vi "Process Event Data.vi"(9 "Event Data":u8[](array[numeric]), 10 "Event Type":u32 format="%.0x", 11 "PS4 Controller in":refnum<class "PS4 Controller.lvclass">) -> (3 "PS4 Controller out":refnum<class "PS4 Controller.lvclass">)   [LabVIEW 2019, in "SDL2 Utility.lvlib" / "PS4 Controller.lvclass"]
uses:
  PS4 Controller.lvclass
  PS4 Controller.lvclass/PS4 Controller.ctl
  LibSDL2 Wrapper/LibSDL2.lvlib
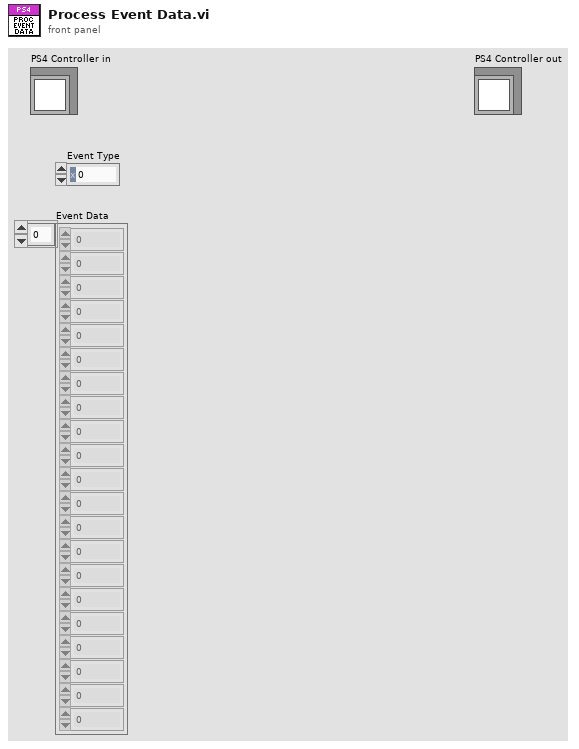
[diagram p1: front panel]
types:
  T1 = typedef "LibSDL2.lvlib/Joysitck Axis Event.ctl" = cluster{"Type":u32, "Timestamp":u32, "Which":i32, "Axis":u8, "Padding 1":u8, "Padding 2":u8, "Padding 3":u8, "Value":i16, "Padding 4":u16}
  T2 = typedef "LibSDL2.lvlib/Joysitck Hat Event.ctl" = cluster{"Type":u32, "Timestamp":u32, "Which":i32, "Hat":u8, "Position":T3}
  T3 = typedef "LibSDL2.lvlib/Joystick Hat Value.ctl" = enum16{"Centred", "Up", "Right", "Down", "Left", "Right Up", "Right Down", "Left Up", "Left Down"}
  T4 = typedef "LibSDL2.lvlib/Joysitck Button Event.ctl" = cluster{"Type":u32, "Timestamp":u32, "Which":i32, "Button":u8, "State":u8, "Padding 1":u8, "Padding 2":u8}
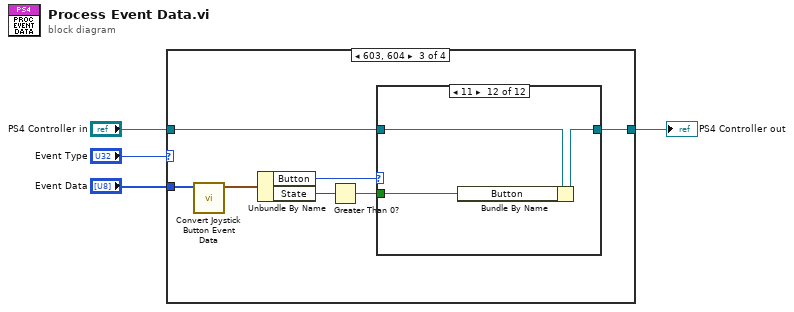
[diagram p0: block diagram]
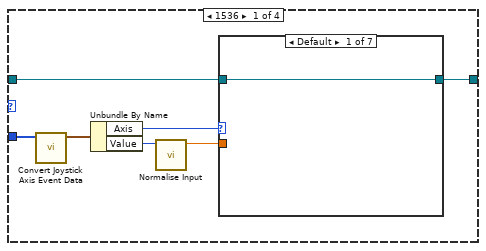
[diagram p2: hidden frame]
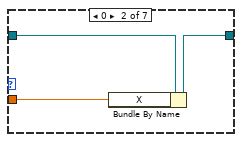
[diagram p3: hidden frame]
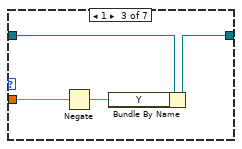
[diagram p4: hidden frame]
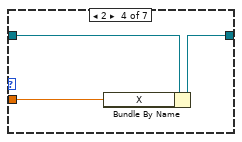
[diagram p5: hidden frame]
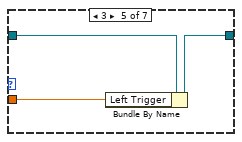
[diagram p6: hidden frame]
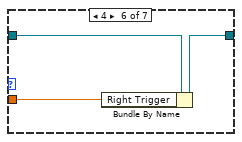
[diagram p7: hidden frame]
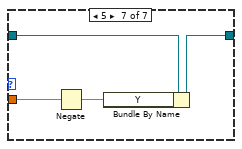
[diagram p8: hidden frame]
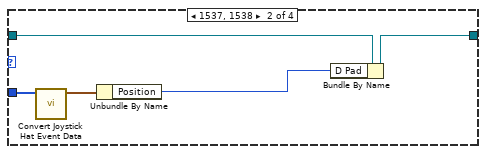
[diagram p9: hidden frame]
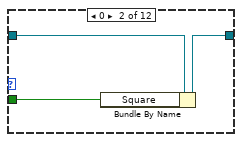
[diagram p11: hidden frame]
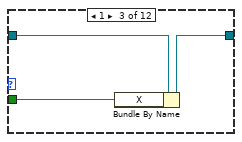
[diagram p12: hidden frame]
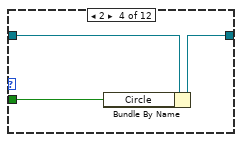
[diagram p13: hidden frame]
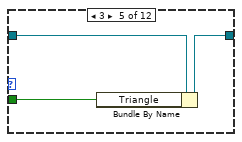
[diagram p14: hidden frame]
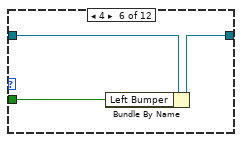
[diagram p15: hidden frame]
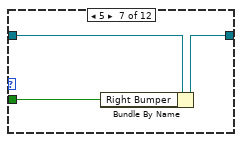
[diagram p16: hidden frame]
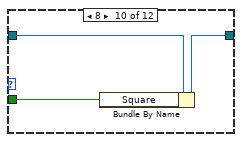
[diagram p19: hidden frame]
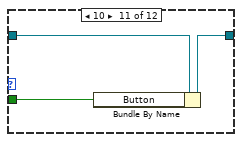
[diagram p20: hidden frame]
diagram:
  n1 = case shown="603, 604" "Event Type" {
    tunnel: "PS4 Controller in" -> [w9 w37 w44 w75]
    tunnel: [w8 w36 w43 w75] -> w2
    tunnel: "Event Data" -> [w7 w35 w42 _]
    frame 1536 {
      n2 = call "Convert Joystick Axis Event Data.vi"("Event Data"=w7) -> ("Joystick Axis Event"=w11:T1)  [unwired: 10 in]
      n3 = Unbundle By Name(w11) -> ("Axis"=w10:u8, "Value"=w6:i16)
      n4 = call "Normalise Input.vi"("Value"=w6) -> ("Value (Normalised)"=w5:sgl)  [unwired: 10 in]
      n5 = case shown="Default" w10 {
        tunnel: w9 -> [w12 w15 w19 w22 w25 w28 w32]
        tunnel: [w12 w14 w18 w21 w24 w27 w31] -> w8
        tunnel: w5 -> [_ w13 w17 w20 w23 w26 w30]
        frame Default {
        }
        frame 0 {
          n6 = Bundle By Name(cluster=w15, "X"=w13) -> (w14:refnum<class "PS4 Controller.lvclass">)
        }
        frame 1 {
          n7 = Negate(x=w17) -> (-x=w16:sgl)
          n8 = Bundle By Name(cluster=w19, "Y"=w16) -> (w18:refnum<class "PS4 Controller.lvclass">)
        }
        frame 2 {
          n9 = Bundle By Name(cluster=w22, "X"=w20) -> (w21:refnum<class "PS4 Controller.lvclass">)
        }
        frame 3 {
          n10 = Bundle By Name(cluster=w25, "Left Trigger"=w23) -> (w24:refnum<class "PS4 Controller.lvclass">)
        }
        frame 4 {
          n11 = Bundle By Name(cluster=w28, "Right Trigger"=w26) -> (w27:refnum<class "PS4 Controller.lvclass">)
        }
        frame 5 {
          n12 = Negate(x=w30) -> (-x=w29:sgl)
          n13 = Bundle By Name(cluster=w32, "Y"=w29) -> (w31:refnum<class "PS4 Controller.lvclass">)
        }
      }
    }
    frame 1537, 1538 {
      n14 = call "Convert Joystick Hat Event Data.vi"("Event Data"=w35) -> ("Joystick Hat Event"=w34:T2)  [unwired: 10 in]
      n15 = Unbundle By Name(w34) -> ("Position"=w33:T3)
      n16 = Bundle By Name(cluster=w37, "D Pad"=w33) -> (w36:refnum<class "PS4 Controller.lvclass">)
    }
    frame 1539, 1540 {
      n17 = call "Convert Joystick Button Event Data.vi"("Event Data"=w42) -> ("Joystick Button Event"=w41:T4)  [unwired: 10 in]
      n18 = Unbundle By Name(w41) -> ("Button"=w40:u8, "State"=w39:u8)
      n19 = Greater Than 0?(x=w39) -> (x > 0?=w38:bool)
      n20 = case shown="11" w40 {
        tunnel: w44 -> [w45 w48 w51 w54 w57 w60 w63 w64 w65 w68 w71 w74]
        tunnel: [w45 w47 w50 w53 w56 w59 w62 w64 w65 w67 w70 w73] -> w43
        tunnel: w38 -> [_ w46 w49 w52 w55 w58 w61 _ _ w66 w69 w72]
        frame Default {
        }
        frame 0 {
          n21 = Bundle By Name(cluster=w48, "Square"=w46) -> (w47:refnum<class "PS4 Controller.lvclass">)
        }
        frame 1 {
          n22 = Bundle By Name(cluster=w51, "X"=w49) -> (w50:refnum<class "PS4 Controller.lvclass">)
        }
        frame 2 {
          n23 = Bundle By Name(cluster=w54, "Circle"=w52) -> (w53:refnum<class "PS4 Controller.lvclass">)
        }
        frame 3 {
          n24 = Bundle By Name(cluster=w57, "Triangle"=w55) -> (w56:refnum<class "PS4 Controller.lvclass">)
        }
        frame 4 {
          n25 = Bundle By Name(cluster=w60, "Left Bumper"=w58) -> (w59:refnum<class "PS4 Controller.lvclass">)
        }
        frame 5 {
          n26 = Bundle By Name(cluster=w63, "Right Bumper"=w61) -> (w62:refnum<class "PS4 Controller.lvclass">)
        }
        frame 6 {
          # "Left Trigger also registers as a button press"
        }
        frame 7 {
          # "Right Trigger also registers as a button press"
        }
        frame 8 {
          n27 = Bundle By Name(cluster=w68, "Square"=w66) -> (w67:refnum<class "PS4 Controller.lvclass">)
        }
        frame 10 {
          n28 = Bundle By Name(cluster=w71, "Button"=w69) -> (w70:refnum<class "PS4 Controller.lvclass">)
        }
        frame 11 {
          n29 = Bundle By Name(cluster=w74, "Button"=w72) -> (w73:refnum<class "PS4 Controller.lvclass">)
        }
      }
    }
    frame Default {
    }
  }
  "PS4 Controller out" <- w2
